vi "TempMain.vi"() -> ()   [LabVIEW 2011]
uses:
  GlobalVariables.vi
  Controls/MFC Cluster.ctl
  Controls/RTPC Cluster.ctl
panel:
  in  "Write Enabled":bool
  in  "Reinitialize?":bool
  in  "stop":bool
  out "RTPC Array":T1[](array[typedef])
  out "Ain":dbl[](array[numeric])
  out "Aout":i16[](array[numeric])
  out "MFC Array":T2[](array[typedef]) {"SetPoint (SCCM)" format="%#.3g"; "Flow (SCCM)" format="%#.4g"}
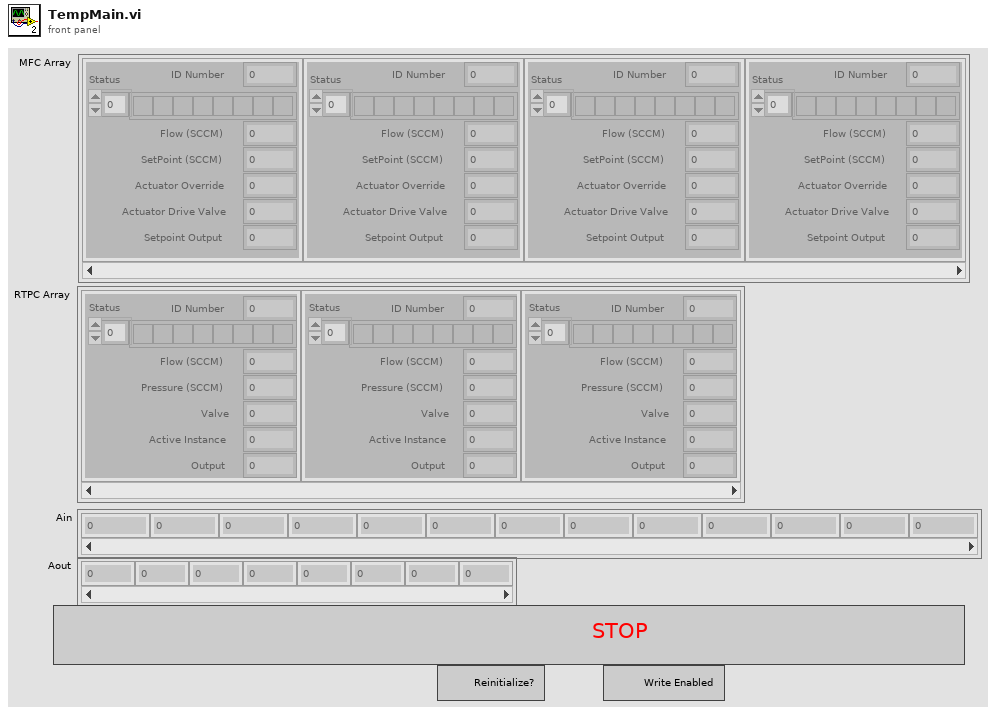
[diagram p1: front panel]
types:
  T1 = typedef "RTPC Cluster.ctl" = cluster{"ID Number":u8, "Status":bool[], "Flow (SCCM)":dbl, "Pressure (SCCM)":dbl, "Valve":i16, "Active Instance":i8, "Output":dbl}
  T2 = typedef "MFC Cluster.ctl" = cluster{"ID Number":u8, "Status":bool[], "Flow (SCCM)":dbl, "SetPoint (SCCM)":dbl, "Actuator Override":i8, "Actuator Drive Valve":i16, "Setpoint Output":dbl}
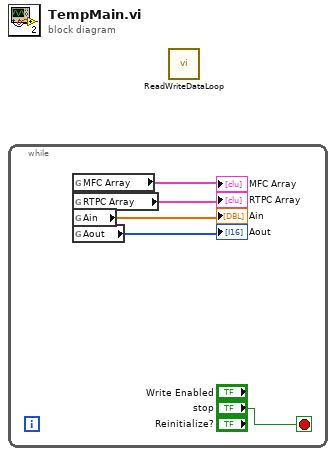
[diagram p0: block diagram]
diagram:
  n1 = while {
    stop <- "stop" stop-if-true
    n2 = global read "GlobalVariables.vi" "MFC Array"() -> (→"MFC Array":T2[])
    n3 = global read "GlobalVariables.vi" "RTPC Array"() -> (→"RTPC Array":T1[])
    n4 = global read "GlobalVariables.vi" "Ain"() -> (→"Ain":dbl[])
    n5 = global read "GlobalVariables.vi" "Aout"() -> (→"Aout":i16[])
  }
  n6 = call "ReadWriteDataLoop.vi"() -> ()  [unwired: 11 in, 1 out]
